vi "SVFA Zoom Cross Spectrum (Mag-Phase).vi"(0 "scaled signal X [EUx]":waveform(dbl)={"t0"=timestamp(0 s since 1904-01-01), "dt"=1e-05, "Y"=[]}, 1 "scaled signal Y [EUy]":waveform(dbl)={"t0"=timestamp(0 s since 1904-01-01), "dt"=1e-05, "Y"=[]}, 3 "zoom settings":T7={"frequency range"={"start frequency"=1000.0, "stop frequency"=2000.0}, "window"=1, "number of lines"=400, "% overlap"=0.0} {"% overlap" min=0.0 format="%.2f"; "number of lines" min=2; "window" items=["None ", "Hanning", "Hamming", "Blackman-Harris", "Exact Blackman", "Blackman", "Flat Top", "4 Term B-Harris ", "7 Term B-Harris", "Low Sidelobe"]; "frequency range"."stop frequency" min=0.0 format="%.2f"; "frequency range"."start frequency" min=0.0 format="%.2f"}, 4 "view":T8={"dB On (T)"=TRUE, "unwrap phase (F)"=FALSE, "convert to degree (T)"=TRUE}, 5 "error in (no error)":errorcluster, 7 "averaging parameters":T9={"averaging mode"=enum."No averaging", "weighting mode"=enum."Exponential", "number of averages"=10, "linear mode"=enum."One shot"} {"number of averages" min=1 step=1}, 9 "restart averaging (F)":bool) -> (11 "averaging done":bool, 12 "new spectrum available":bool, 13 "averages completed":dbl, 14 "magnitude [dB EUx EUy]":cluster{"f0":dbl, "df":dbl, "magnitude":dbl[]} {"magnitude" format="%.2p"; "df" format="%.2p"; "f0" format="%.2p"}, 15 "magnitude unit label":string, 16 "phase [degrees]":cluster{"f0":dbl, "df":dbl, "phase":dbl[]} {"phase" format="%.2f"; "df" format="%.2f"; "f0" format="%.2f"}, 17 "phase unit label":string, 18 "spectrum info":T1={"channel name"="", "description"="", "x-axis units"=1, "spectral info"={"spectrum type"=enum."Power [Magnitude^2]", "linear/dB"=enum."linear", "window"=0, "window size"=0, "FFT size"=0}, "engineering units"=0, "custom label"="", "dB reference [EU]"=0.0, "peak units"=enum."rms", "weighting filter"=0, "spectral density?"=FALSE, "unit label"="", "spectrum skewed?"=FALSE, "complimentary spectrum units"=enum."none"} {"x-axis units" items=["Time (s)"=0, "Frequency-CB (Hz)"=1, "Frequency-CPB (Hz)"=1248, "Frequency-Arbitrary (Hz)"=2357, "Quefrency (s)"=2, "Revolutions (rev)"=3, "Order"=4, "Speed (RPM)"=11, "Speed (rad/s)"=21, "Index"=65535]; "weighting filter" items=["Linear", "A-weighting", "B-weighting", "C-weighting", "ITU-R 468-4", "Dolby", "CCITT", "C-message", "Wb", "Wc", "Wd", "We", "Wf", "Wh", "Wj", "Wk", "Wm", "AES17 20 kHz lowpass", "AES17 40 kHz lowpass", "AES17 20 kHz highpass", "AES17 40 kHz highpass"]; "dB reference [EU]" format="%.2f"; "engineering units" items=["custom..."=0, "V"=1, "A"=21, "C"=30, "pC"=31, "s"=32, "-"=29, "Pa"=2, "N"=20, "g"=3, "m/s^2"=4, "m/s"=5, "m"=6, "mm/s"=12, "mm"=13, "micron/s"=14, "micron"=15, "in/s^2"=7, "in/s"=8, "in"=9, "mil/s"=10, "mil"=11, "rad/s^2"=16, "rad/s"=17, "rad"=18, "deg/s^2"=26, "deg/s"=27, "deg"=28, "RPM"=22, "cycle/s^2"=23, "Hz"=24, "cycle"=25, "strain"=19]; "spectral info"."window" items=["None "=0, "Hanning"=1, "Hamming"=2, "Blackman-Harris"=3, "Exact Blackman"=4, "Blackman"=5, "Flat Top"=6, "4 Term B-Harris "=7, "7 Term B-Harris"=8, "Low Sidelobe"=9, "Force - Exponential"=10, "Gaussian"=62]}, 19 "error out":errorcluster)   [LabVIEW 2017]
doc: "Computes the zoom cross power spectrum of <B>scaled signal X [EUx]</B>, <B>scaled signal Y [EUy]</B>, and <B>zoom settings</B>. Results are returned in magnitude and phase. Data accumulates each time the VI is called. However, it returns a new spectrum only when sufficient data accumulates. Indicators and subsequent processing should only be called when <B>new spectrum available</B> is TRUE."
uses:
  <vilib>/addons/_NISVFA/_Shared subVIs/Controls/svc_Spectrum Info.ctl
  <vilib>/addons/_NISVFA/_Shared subVIs/Controls/svc_X-Axis Units.ctl
  <vilib>/addons/_NISVFA/_Shared subVIs/Controls/svc_Spectrum Type.ctl
  <vilib>/addons/_NISVFA/_Shared subVIs/Controls/svc_Engineering Units Text Ring.ctl
  <vilib>/addons/_NISVFA/_Shared subVIs/Controls/svc_Weighting Filter Text Ring.ctl
  <vilib>/addons/_NISVFA/_Shared subVIs/Controls/svc_Complimentary Spectrum Units.ctl
  <vilib>/addons/_NISVFA/_Shared subVIs/Spectrum Averaging/svfa_Reset Averaging State Info.vi
  <vilib>/addons/_NISVFA/_Shared subVIs/Spectrum Averaging/svfa_Average Array with Avg Checks (complex) No State.vi
  <vilib>/addons/_NISVFA/_Shared subVIs/Spectrum Averaging/svfa_Average Array (complex) No State.vi
  <vilib>/addons/_NISVFA/_Shared subVIs/Spectrum Averaging/svfa_No Average Array (complex).vi
  <vilib>/addons/_NISVFA/_Shared subVIs/Spectrum Averaging/svfa_Average Array (complex).vi
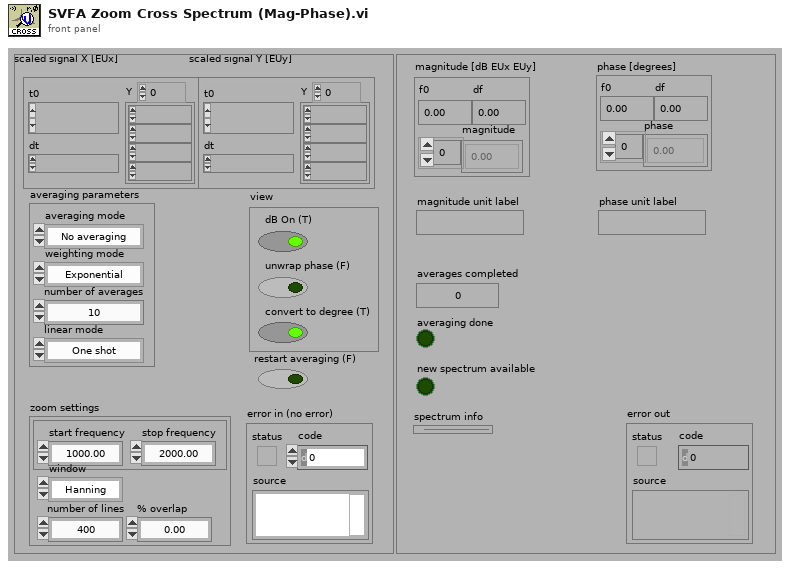
[diagram p1: front panel]
types:
  T1 = typedef "svc_Spectrum Info.ctl" = cluster{"channel name":string, "description":string, "x-axis units":T2, "spectral info":cluster{"spectrum type":T3, "linear/dB":enum16{"linear", "dB"}, "window":u16, "window size":i32, "FFT size":i32}, "engineering units":T4, "custom label":string, "dB reference [EU]":dbl, "peak units":enum16{"rms", "peak", "peak-peak"}, "weighting filter":T5, "spectral density?":bool, "unit label":string, "spectrum skewed?":bool, "complimentary spectrum units":T6}
  T2 = typedef "svc_X-Axis Units.ctl" = u16
  T3 = typedef "svc_Spectrum Type.ctl" = enum16{"FFT Spectrum [complex]", "Amplitude [Magnitude]", "Power [Magnitude^2]", "Cross Spectrum [complex]", "Frequency Response [Complex]"}
  T4 = typedef "svc_Engineering Units Text Ring.ctl" = u16
  T5 = typedef "svc_Weighting Filter Text Ring.ctl" = u16
  T6 = typedef "svc_Complimentary Spectrum Units.ctl" = enum16{"none", "radians", "degrees", "cycles", "imaginary"}
  T7 = cluster{"frequency range":cluster{"start frequency":dbl, "stop frequency":dbl}, "window":u16, "number of lines":i32, "% overlap":dbl}
  T8 = cluster{"dB On (T)":bool, "unwrap phase (F)":bool, "convert to degree (T)":bool}
  T9 = cluster{"averaging mode":enum16{"No averaging", "Vector averaging", "RMS averaging", "Peak hold"}, "weighting mode":enum16{"Linear", "Exponential"}, "number of averages":u32, "linear mode":enum16{"One shot", "Auto restart"}}
  T10 = enum16{"Restart processing", "Continue processing", "Skip processing"}
  T11 = enum16{"Cross spectrum", "Frequency response", "Coherent output power"}
  T12 = enum16{"No averaging", "Vector averaging", "RMS averaging", "Peak hold"}
  T13 = cluster{"zoom settings":cluster{"center frequency":dbl, "zoom":i32, "trim":dbl}, "FFT settings":cluster{"window":enum16{"None ", "Hanning", "Hamming", "Blackman-Harris", "Exact Blackman", "Blackman", "Flat Top", "4 Term B-Harris ", "7 Term B-Harris", "Low Sidelobe"}, "window size":i32, "FFT size":i32, "%overlap":dbl}}
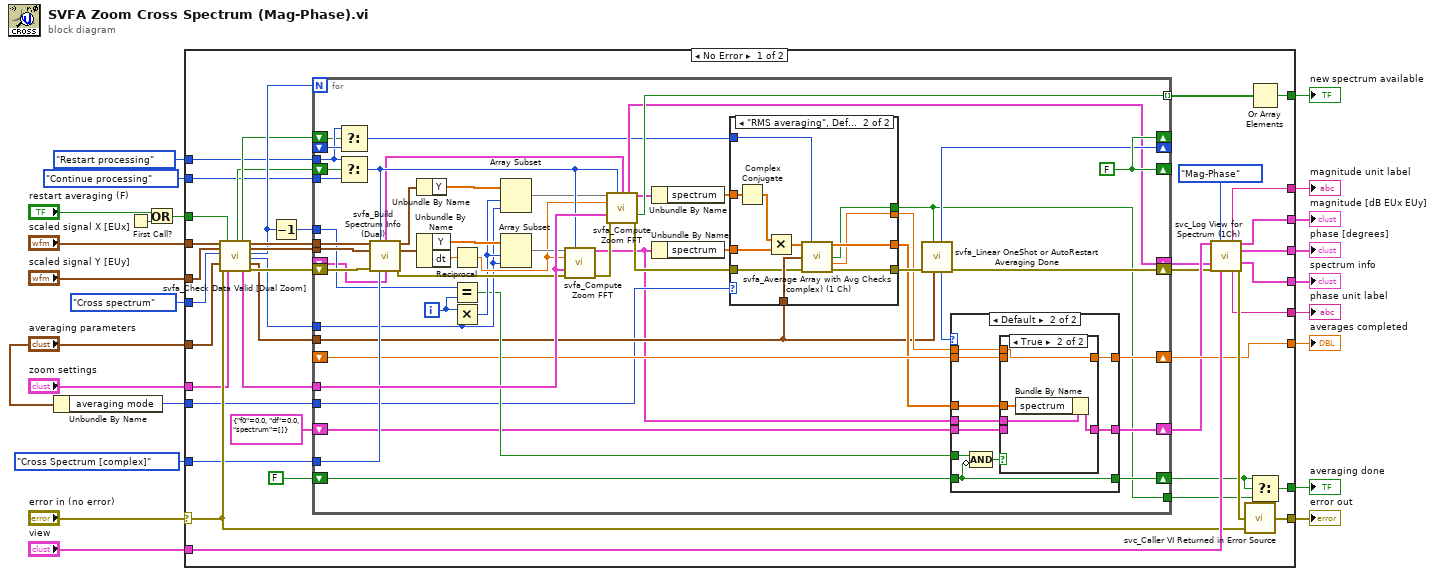
[diagram p0: block diagram]
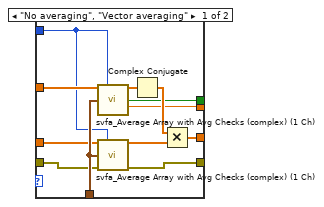
[diagram p2: hidden frame]
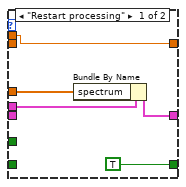
[diagram p3: hidden frame]
diagram:
  n1 = Unbundle By Name("averaging parameters") -> ("averaging mode"=w13:T12)
  n2 = First Call?() -> (First Call?: T/F=w23:bool)
  n3 = Or(x="restart averaging (F)", y=w23) -> (x .or. y?=w17:bool)
  n4 = case shown="No Error" "error in (no error)" {
    selector: "error in (no error)" -> [w52 w160]
    tunnel: "scaled signal X [EUx]" -> [w64 _]
    tunnel: "scaled signal Y [EUy]" -> [w63 _]
    tunnel: [w60 _] -> w4
    tunnel: [w59 _] -> w5
    tunnel: [w53 w160] -> w7
    tunnel: [w25 _] -> w3
    tunnel: w17 -> [w61 _]
    tunnel: "view" -> [w57 _]
    tunnel: "zoom settings" -> [w50 _]
    tunnel: [w27 _] -> w11
    tunnel: [w47 _] -> w10
    tunnel: [w58 _] -> w6
    tunnel: [w56 _] -> w9
    tunnel: [w54 _] -> w8
    tunnel: "averaging parameters" -> [w62 _]
    tunnel: T11."Cross spectrum" ("measurement") -> [w49 _]
    tunnel: svc_Spectrum_Type."Cross Spectrum [complex]" ("spectrum type") -> [w36 _]
    tunnel: w13 -> [w35 _]
    tunnel: T10."Restart processing" ("processing control") -> [w32 _]
    tunnel: T10."Continue processing" ("processing control") -> [w31 _]
    frame No Error {
      n5 = call <vilib>:"svfa_Check Data Valid [Dual Zoom].vi"("stimulus [X]"=w64, "response [Y]"=w63, "measurement"=w49, "averaging parameters"=w62, "error in (no error)"=w52, "restart averaging (F)"=w61, "zoom settings"=w50) -> ("reset processing"=w33:bool, "restart averaging"=w34:bool, "zoom FFT settings"=w37:T13, "dup stimulus [X]"=w43:waveform(dbl), "dup response [Y]"=w42:waveform(dbl), "iterations"=w39:i32, "maximum block size"=w30:i32, "dup averaging parameters"=w40:T9, "error out"=w41:errorcluster)  [unwired: 3 in, 1 out]
      n6 = Decrement(x=w39) -> (x-1=w38:i32)
      n7 = for {
        N: w39 -> [_]
        shift-left: cluster{"f0":dbl, "df":dbl, "spectrum":cdb[]} {"f0"=0.0, "df"=0.0, "spectrum"=[]} ("FFT spectrum") -> [w81]
        shift-right: [w82] -> w46
        tunnel: w40 -> [w70]
        tunnel: [w72] -> w24
        tunnel: [w80] -> w48 mode=indexing
        tunnel: w42 -> [w110]
        tunnel: w43 -> [w111]
        shift-right: [w78] -> w45
        shift-left: _ -> [w77]
        shift-right: [w88] -> _
        shift-left: _ -> [w102]
        tunnel: w38 -> [w96]
        tunnel: w37 -> [w114]
        tunnel: w36 -> [w105]
        tunnel: w35 -> [w69]
        shift-right: [w115] -> w44
        shift-left: w41 -> [w106]
        shift-right: [w84] -> w47
        shift-left: _ -> [w83]
        shift-right: [w98] -> _
        shift-left: w34 -> [w100]
        shift-right: [w98] -> _
        shift-left: w33 -> [w104]
        tunnel: w32 -> [w101]
        tunnel: w31 -> [w103]
        tunnel: w30 -> [w89]
        shift-right: [w86] -> w26
        shift-left: FALSE ("restart averaging") -> [w85]
        i -> [w97]
        w98 = FALSE ("reset processing")
        n8 = Select(t=w101, s=w100, f=w102) -> (s? t:f=w76:T10)
        n9 = Select(t=w101, s=w104, f=w103) -> (s? t:f=w99:T10)
        n10 = call <vilib>:"svfa_Build Spectrum Info (Dual).vi"("scaled signal  X [EU]"=w111, "processing control"=w99, "scaled signal  Y [EU]"=w110, "error in (no error)"=w106, "spectrum type"=w105, "spectrum info in"=w77) -> ("spectrum info out"=w79:T1, "dup scaled signal  X [EU]"=w109:waveform(dbl), "dup scaled signal  Y [EU]"=w108:waveform(dbl), "error out"=w107:errorcluster)  [unwired: 5 in, 1 out]
        n11 = Unbundle By Name ("Get Waveform Components")(w109) -> ("Y"=w95:dbl[])
        n12 = Unbundle By Name ("Get Waveform Components")(w108) -> ("Y"=w93:dbl[], "dt"=w113:dbl)
        n13 = Reciprocal(x=w113) -> (1/x=w91:dbl)
        n14 = Equal?(x=w96, y=w97) -> (x = y?=w87:bool)
        n15 = Multiply(x=w97, y=w89) -> (x*y=w90:i32)
        n16 = Array Subset(array=w95, index=w90, length=w89) -> (w94:dbl[])
        n17 = Array Subset(array=w93, index=w90, length=w89) -> (w92:dbl[])
        n18 = call <vilib>:"svfa_Compute Zoom FFT.vi"("x"=w92, "processing control"=w99, "fs"=w91, "zoom FFT settings"=w114, "error in (no error)"=w107) -> ("FFT spectrum"=w68:cluster{"f0":dbl, "df":dbl, "spectrum":cdb[]}, "error out"=w112:errorcluster)  [unwired: 6 in, 3 out]
        n19 = call <vilib>:"svfa_Compute Zoom FFT.vi"("x"=w94, "processing control"=w99, "spectrum info"=w79, "fs"=w91, "zoom FFT settings"=w114, "error in (no error)"=w112) -> ("spectrum info out"=w78:T1, "FFT spectrum"=w66:cluster{"f0":dbl, "df":dbl, "spectrum":cdb[]}, "spectrum ready"=w80:bool, "error out"=w75:errorcluster)  [unwired: 5 in, 1 out]
        n20 = Unbundle By Name(w66) -> ("spectrum"=w65:cdb[])
        n21 = Unbundle By Name(w68) -> ("spectrum"=w67:cdb[])
        n22 = case shown="\"RMS averaging\", Default" w69 {
          tunnel: [w118 w134] -> w71
          tunnel: [w119 w135] -> w72
          tunnel: w70 -> [w122 w132]
          tunnel: w65 -> [w121 w129]
          tunnel: w67 -> [w120 w128]
          tunnel: [w126 w136] -> w73
          tunnel: w75 -> [w117 w131]
          tunnel: [w123 w130] -> w74
          tunnel: w76 -> [w116 w133]
          frame "No averaging", "Vector averaging" {
            n23 = call <vilib>:"svfa_Average Array with Avg Checks (complex) (1 Ch).vi"("spectrum"=w121, "processing control"=w116, "averaging parameters"=w122) -> ("average spectrum"=w125:cdb[], "averaging done"=w119:bool, "averages completed"=w118:dbl)  [unwired: 8 in, 2 out]
            n24 = call <vilib>:"svfa_Average Array with Avg Checks (complex) (1 Ch).vi"("spectrum"=w120, "processing control"=w116, "averaging parameters"=w122, "error in (no error)"=w117) -> ("average spectrum"=w124:cdb[], "error out"=w123:errorcluster)  [unwired: 7 in, 3 out]
            n25 = Complex Conjugate(1:w125) -> (0:w127:cdb[])
            n26 = Multiply(x=w127, y=w124) -> (x*y=w126:cdb[])
          }
          frame "RMS averaging", Default {
            n27 = Complex Conjugate(1:w129) -> (0:w138:cdb[])
            n28 = Multiply(x=w138, y=w128) -> (x*y=w137:cdb[])
            n29 = call <vilib>:"svfa_Average Array with Avg Checks (complex) (1 Ch).vi"("spectrum"=w137, "processing control"=w133, "averaging parameters"=w132, "error in (no error)"=w131) -> ("average spectrum"=w136:cdb[], "averaging done"=w135:bool, "averages completed"=w134:dbl, "error out"=w130:errorcluster)  [unwired: 7 in, 1 out]
          }
        }
        n30 = call <vilib>:"svfa_Linear OneShot or AutoRestart Averaging Done.vi"("averaging parameters"=w70, "averaging done"=w72, "error in (no error)"=w74) -> ("error out"=w115:errorcluster, "processing control"=w88:T10)  [unwired: 7 in]
        n31 = case shown="Default" w88 {
          tunnel: [TRUE ("restart averaging") w151] -> w86
          tunnel: w85 -> [_ w151]
          tunnel: w87 -> [_ w153]
          tunnel: [w142 w150] -> w84
          tunnel: w83 -> [_ w149]
          tunnel: w71 -> [w142 w148]
          tunnel: w68 -> [w139 w144]
          tunnel: w73 -> [w141 w146]
          tunnel: [w140 w147] -> w82
          tunnel: w81 -> [_ w145]
          frame "Restart processing" {
            n32 = Bundle By Name(cluster=w139, "spectrum"=w141) -> (w140:cluster{"f0":dbl, "df":dbl, "spectrum":cdb[]})
          }
          frame Default {
            n33 = Compound Arithmetic op=AND(w153, invert w151) -> (w152:bool)
            n34 = case shown="True" w152 {
              tunnel: [w155 w159] -> w150
              tunnel: w149 -> [w155 _]
              tunnel: w148 -> [_ w159]
              tunnel: w144 -> [_ w156]
              tunnel: [w154 w158] -> w147
              tunnel: w146 -> [_ w157]
              tunnel: w145 -> [w154 _]
              frame False {
              }
              frame True {
                n35 = Bundle By Name(cluster=w156, "spectrum"=w157) -> (w158:cluster{"f0":dbl, "df":dbl, "spectrum":cdb[]})
              }
            }
          }
        }
      }
      n36 = call <vilib>:"svc_Log View for Spectrum (1Ch).vi"("complex spectrum"=w46, "View"=enum16{"Mag-Phase", "Real-Imaginary"}."Mag-Phase", "spectrum info in"=w45, "error in (no error)"=w44, "view"=w57) -> ("unit label [mag or real]"=w56:string, "magnitude or real"=w60:cluster{"f0":dbl, "df":dbl, dbl[]}, "phase or imag"=w59:cluster{"f0":dbl, "df":dbl, dbl[]}, "spectrum info out"=w58:T1, "unit label [phase or imag]"=w54:string, "error out"=w55:errorcluster)  [unwired: 5 in]
      n37 = call <vilib>:"svc_Caller VI Returned in Error Source.vi"("warning input to caller"=w52, "error in (no error)"=w55) -> ("error out"=w53:errorcluster)  [unwired: 3 in]
      n38 = Or Array Elements(Boolean array=w48) -> (logical OR=w27:bool)
      n39 = Select(t=w26, s=w26, f=w24) -> (s? t:f=w25:bool)
    }
    frame Error {
    }
  }
  "error out" <- w7
  "phase [degrees]" <- w5
  "magnitude [dB EUx EUy]" <- w4
  "magnitude unit label" <- w9
  "phase unit label" <- w8
  "averages completed" <- w10
  "averaging done" <- w3
  "new spectrum available" <- w11
  "spectrum info" <- w6
